vi "Get or Create Action Point.vi"(8 "Error In":errorcluster, 10 "Action Point Identifier":string) -> (0 "Error Out":errorcluster, 2 "IAction Point":refnum<class "IVirtual Instrument.lvclass">)   [LabVIEW 2024, in "Instrument Manager.lvclass"]
uses:
  Instrument Manager.lvclass
  Interfaces/IVirtual Instrument/IVirtual Instrument.lvclass
  Action Point/Action Point.lvclass
  Instrument Manager.lvclass/Instrument Manager.ctl
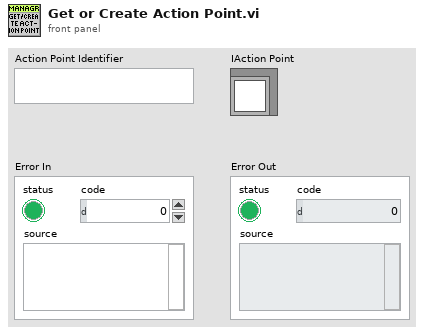
[diagram p1: front panel]
types:
  T1 = map{string, refnum<class "Action Point.lvclass">}
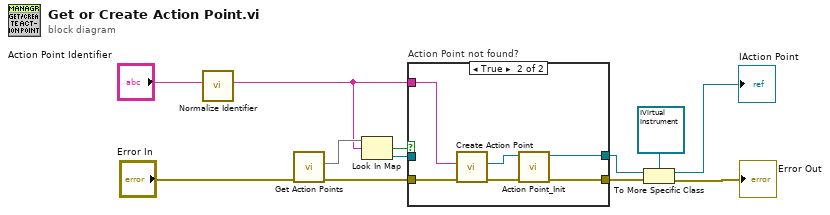
[diagram p0: block diagram]
diagram:
  n1 = call "Normalize Identifier.vi"("Identifier"="Action Point Identifier") -> ("Normalized Identifier"=w1:string)  [unwired: 10 in]
  n2 = call "Get Action Points.vi"("Error In"="Error In") -> ("Error Out"=w8:errorcluster, "Action Points"=w7:T1)  [unwired: 9 in]
  n3 = Look In Map(map=w7, key=w1) -> (key not found?=w6:bool, value=w5:refnum<class "Action Point.lvclass">)  [unwired: 1 in]
  n4 = case "Action Point not found?" shown="True" w6 {
    tunnel: [w14 w17] -> w3
    tunnel: w8 -> [w14 w19]
    tunnel: w5 -> [w13 _]
    tunnel: [w13 w16] -> w2
    tunnel: w1 -> [_ w15]
    frame False {
    }
    frame True {
      n5 = call "Create Action Point.vi"("error in"=w19, "Action Point Identifier"=w15) -> ("error out"=w20:errorcluster, "IAction Point out"=w18:refnum<class "Action Point.lvclass">)  [unwired: 8 in]
      n6 = call-dynamic "Action Point_Init.vi"("error in"=w20, "Action Point in"=w18) -> ("error out"=w17:errorcluster, "Action Point out"=w16:refnum<class "Action Point.lvclass">)  [unwired: 8 in]
    }
  }
  n7 = To More Specific Class(target class=refnum<class "IVirtual Instrument.lvclass"> refnum ("IVirtual Instrument.lvclass"), reference=w2, error in=w3) -> (specific class reference=→"IAction Point":refnum<class "IVirtual Instrument.lvclass">, error out=→"Error Out":errorcluster)
